vi "截取字符串(除2).vi"(3 "长度":i32[](array[numeric]), 4 "数组 2":i32[](array[numeric]), 5 "数组1":i32[](array[numeric])) -> (1 "子数组2":i32[](array[numeric]), 2 "子数组1":dbl[](array[numeric]) format="%.2f")   [LabVIEW 2019]
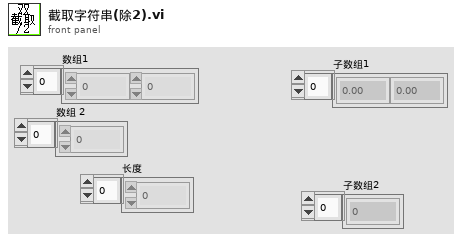
[diagram p1: front panel]
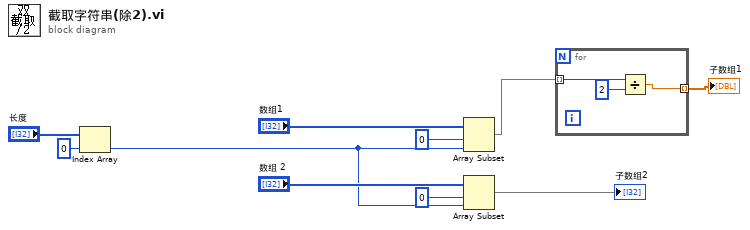
[diagram p0: block diagram]
diagram:
  n1 = Index Array(array="长度", index=0 ("索引")) -> (element=w3:i32)
  n2 = Array Subset(array="数组1", index=0 ("索引"), length=w3) -> (w2:i32[])
  n3 = Array Subset(array="数组 2", index=0 ("索引"), length=w3) -> (→"子数组2":i32[])
  n4 = for {
    tunnel: w2 -> [w13] mode=indexing
    tunnel: [w11] -> w1 mode=indexing
    n5 = Divide(x=w13, y=2) -> (x/y=w11:dbl)
  }
  "子数组1" <- w1
